vi "read sync.vi"(8 "error in (no error)":errorcluster, 9 "len":i32, 10 "buf":u8[](array[numeric]), 11 "DevRefnum":u64) -> (0 "error out":errorcluster, 2 "buf 2":u8[](array[numeric]), 3 "DevRefnum":u64)   [LabVIEW 2013, in "rtlsdr.lvlib"]
doc: "RTLSDR_API int rtlsdr_read_sync(rtlsdr_dev_t *dev, void *buf, int len, int *n_read);"
uses:
  <instrlib>/rtlsdr/rtlsdr.lvlib
  <instrlib>/rtlsdr/VIs/rtlsdr.dll
panel:
  in  "n_read":i32
  out "n_read out":i32
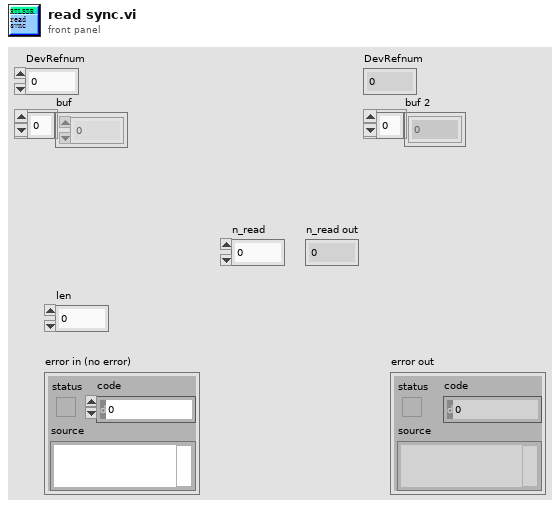
[diagram p1: front panel]
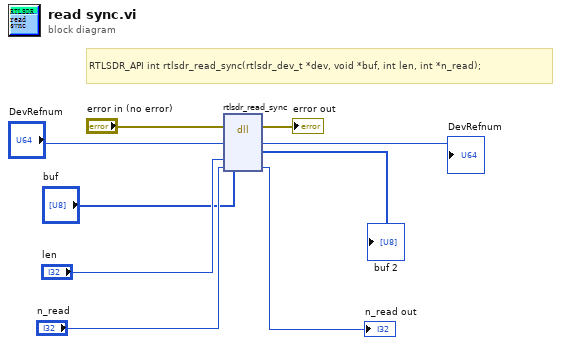
[diagram p0: block diagram]
diagram:
  # "RTLSDR_API int rtlsdr_read_sync(rtlsdr_dev_t *dev, void *buf, int len, int *n_read);"
  n1 = dll-call lib="C:/Program Files (x86)/National Instruments/LabVIEW 2013/instr.lib/rtlsdr/VIs/rtlsdr.*" fn="rtlsdr_read_sync"(error in="error in (no error)", "DevRefnum"="DevRefnum", "buf"="buf", "len"="len", "n_read"="n_read") -> (error out=→"error out":errorcluster, "DevRefnum"=→"DevRefnum":u64, "buf"=→"buf 2":u8[], "n_read"=→"n_read out":i32)  [unwired: 4 in, 1 out]
